vi "lib ReadCSVwithQuotes.vi"(4 "String":string="123,\"test,number1\"\n\"hi, file\",46\n\"you're \"\"fine\"\"\",\"0,4\"\n") -> (1 "Array":string[][](array[string]))   [LabVIEW 2021]
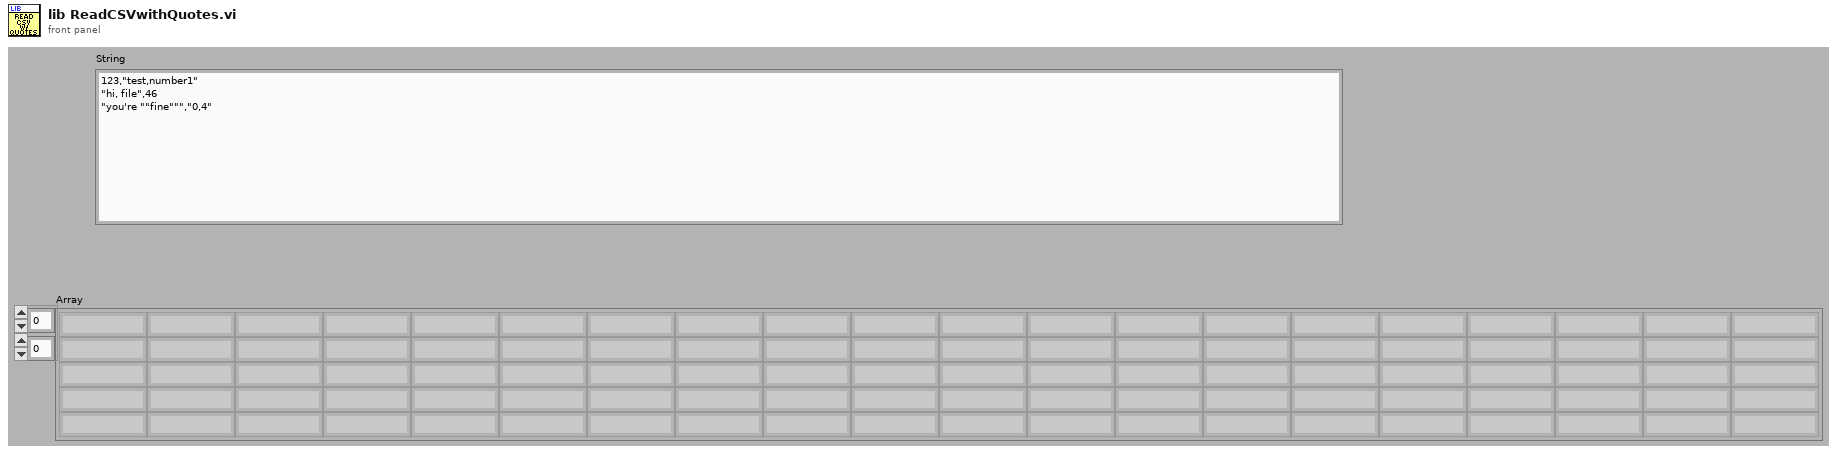
[diagram p1: front panel]
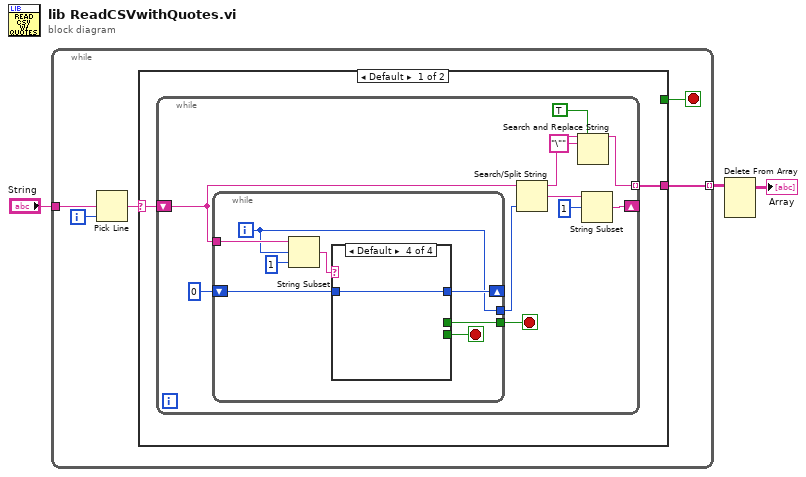
[diagram p0: block diagram]
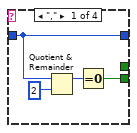
[diagram p2: hidden frame]
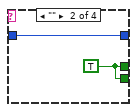
[diagram p3: hidden frame]
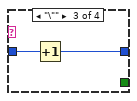
[diagram p4: hidden frame]
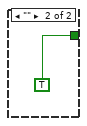
[diagram p5: hidden frame]
diagram:
  n1 = while {
    tunnel: "String" -> [w7]
    tunnel: [w4] -> w2 mode=indexing
    i -> [w8]
    stop <- w5 stop-if-true
    n2 = Pick Line(multi-line string=w7, line index=w8) -> (output string=w6:string)  [unwired: 1 in]
    n3 = case shown="Default" w6 {
      selector: w6 -> [w10 _]
      tunnel: [_ TRUE] -> w5
      tunnel: [w9 _] -> w4
      frame Default {
        n4 = while {
          tunnel: [w13] -> w9 mode=indexing
          shift-right: [w15] -> _
          shift-left: w10 -> [w20]
          stop <- w19 stop-if-true
          n5 = while {
            tunnel: w20 -> [w24]
            shift-right: [w26] -> _
            shift-left: 0 -> [w27]
            tunnel: [w23] -> w19
            tunnel: [w22] -> w18
            i -> [w22]
            stop <- w25 stop-if-true
            n6 = String Subset(string=w24, offset (0)=w22, length (rest)=1 ("length (rest)")) -> (substring=w28:string)
            n7 = case shown="Default" w28 {
              tunnel: w27 -> [w33 w34 w37 w38]
              tunnel: [w33 w34 w36 w38] -> w26
              tunnel: [w30 w35 _ _] -> w25
              tunnel: [_ w35 _ _] -> w23
              frame "," {
                n8 = Quotient & Remainder(x=w33, y=2) -> (x-y*floor(x/y)=w31:i32)  [unwired: 1 out]
                n9 = Equal To 0?(x=w31) -> (x = 0?=w30:bool)
              }
              frame "" {
                w35 = TRUE
              }
              frame "\"" {
                n10 = Increment(x=w37) -> (x+1=w36:i32)
              }
              frame Default {
              }
            }
          }
          n11 = Search/Split String(string=w20, offset (0)=w18) -> (substring before match=w14:string, match + rest of string=w17:string)  [unwired: 1 in, 1 out]
          n12 = Search and Replace String(replace all?=TRUE ("replace all? (F)"), input string=w14, search string="\"") -> (result string=w13:string)  [unwired: 5 in, 3 out]
          n13 = String Subset(string=w17, offset (0)=1) -> (substring=w15:string)  [unwired: 1 in]
        }
      }
      frame "" {
      }
    }
  }
  n14 = Delete From Array(array=w2) -> (array with subset deleted=→"Array":string[][])  [unwired: 3 in, 1 out]
